vi "Last Ack.vi"(10 "Alias":string, 11 "Dev Actor in":refnum<class "Dev Actor.lvclass">) -> (3 "Dev Actor out":refnum<class "Dev Actor.lvclass">)   [LabVIEW 2021, in "Dev Actor.lvlib" / "Dev Actor.lvclass"]
uses:
  Dev Actor.lvclass
  Dev Actor.lvclass/Dev Actor.ctl
  Queue Actor/Queue Actor.lvclass
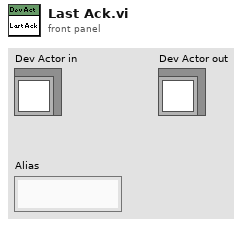
[diagram p1: front panel]
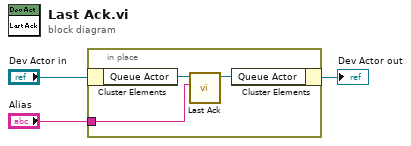
[diagram p0: block diagram]
diagram:
  n1 = in-place {
    in-place-border: "Alias" -> [w4]
    n2 = in-place-cluster #1("Dev Actor in") -> ("Queue Actor"=w5:refnum<class "Queue Actor.lvclass">)
    n3 = call-dynamic "Last Ack.vi"("Alias"=w4, "Last Ack in"=w5) -> ("Last Ack out"=w6:refnum<class "Queue Actor.lvclass">)  [unwired: 9 in]
    n4 = in-place-cluster #1("Queue Actor"=w6) -> (→"Dev Actor out":refnum<class "Dev Actor.lvclass">)
  }
